vi "Run FGV Tests for 2D Double Array.vi"(2 "DELETE VI Reference":refnum<vi>, 3 "GET VI Reference":refnum<vi>, 4 "PUT VI Reference":refnum<vi>) -> (0 "Reason":string, 1 "Success":bool)   [LabVIEW 2013]
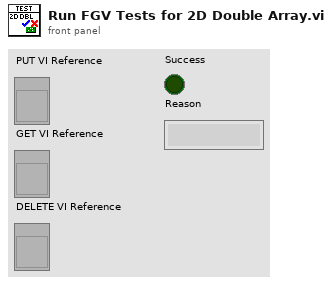
[diagram p1: front panel]
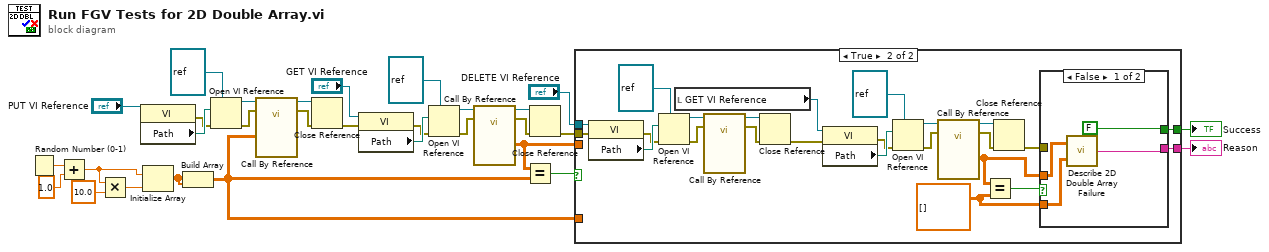
[diagram p0: block diagram]
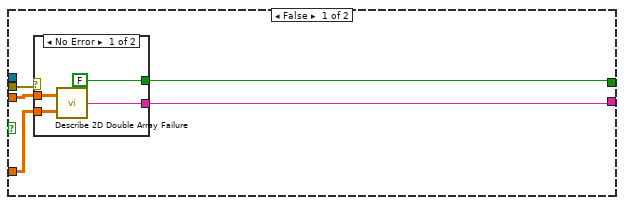
[diagram p2: hidden frame]
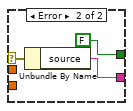
[diagram p3: hidden frame]
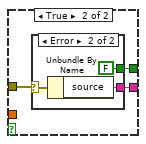
[diagram p4: hidden frame]
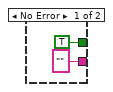
[diagram p5: hidden frame]
diagram:
  n1 = Random Number (0-1)() -> (number: 0 to 1=w15:dbl)
  n2 = Add(x=w15, y=1.0) -> (x+y=w3:dbl)
  n3 = Multiply(x=w3, y=10.0) -> (x*y=w4:dbl)
  n4 = property class="VI"(reference="PUT VI Reference") -> (error out=w8:errorcluster, "Path"=w21:path)  [unwired: 1 in, 1 out]
  n5 = Initialize Array(w3, w4) -> (w2:dbl[])
  n6 = Build Array(w2, w2) -> (w1:dbl[][])
  n7 = Open VI Reference(type specifier VI Refnum (for type only)=refnum<vi> refnum, vi path=w21, error in (no error)=w8) -> (vi reference=w20:refnum<vi>, error out=w19:errorcluster)  [unwired: 3 in]
  n8 = call-by-ref "?"(reference=w20, error in=w19, "Data"=w1) -> (reference out=w18:refnum<vi>, error out=w17:errorcluster)
  n9 = Close Reference(reference=w18, error in (no error)=w17) -> (error out=w13:errorcluster)
  n10 = property class="VI"(reference="GET VI Reference", error in=w13) -> (error out=w9:errorcluster, "Path"=w26:path)  [unwired: 1 out]
  n11 = Open VI Reference(type specifier VI Refnum (for type only)=refnum<vi> refnum, vi path=w26, error in (no error)=w9) -> (vi reference=w27:refnum<vi>, error out=w28:errorcluster)  [unwired: 3 in]
  n12 = call-by-ref "?"(reference=w27, error in=w28) -> (reference out=w29:refnum<vi>, error out=w30:errorcluster, "Data"=w10:dbl[][])
  n13 = Equal?(x=w10, y=w1) -> (x = y?=w11:bool)
  n14 = Close Reference(reference=w29, error in (no error)=w30) -> (error out=w12:errorcluster)
  n15 = case shown="True" w11 {
    tunnel: "DELETE VI Reference" -> [_ w60]
    tunnel: w12 -> [w31 w59]
    tunnel: w1 -> [w34 _]
    tunnel: w10 -> [w35 _]
    tunnel: [w33 w45] -> w7
    tunnel: [w32 w44] -> w6
    frame False {
      n16 = case shown="No Error" w31 {
        selector: w31 -> [_ w42]
        tunnel: w35 -> [w39 _]
        tunnel: w34 -> [w38 _]
        tunnel: [FALSE FALSE] -> w33
        tunnel: [w36 w40] -> w32
        frame No Error {
          n17 = call "Describe 2D Double Array Failure.vi"("Expected"=w38, "Got"=w39) -> ("Failure Description"=w36:string)
        }
        frame Error {
          n18 = Unbundle By Name(w42) -> ("source"=w40:string)
        }
      }
    }
    frame True {
      w43 = dbl[][] [] ("appended array")
      n19 = property class="VI"(reference=w60, error in=w59) -> (error out=w49:errorcluster, "Path"=w62:path)  [unwired: 1 out]
      n20 = Open VI Reference(type specifier VI Refnum (for type only)=refnum<vi> refnum, vi path=w62, error in (no error)=w49) -> (vi reference=w63:refnum<vi>, error out=w64:errorcluster)  [unwired: 3 in]
      n21 = local read "GET VI Reference"() -> (w47:refnum<vi>)
      n22 = call-by-ref "?"(reference=w63, error in=w64) -> (reference out=w65:refnum<vi>, error out=w66:errorcluster)  [unwired: 1 in]
      n23 = Close Reference(reference=w65, error in (no error)=w66) -> (error out=w52:errorcluster)
      n24 = property class="VI"(reference=w47, error in=w52) -> (error out=w50:errorcluster, "Path"=w54:path)  [unwired: 1 out]
      n25 = Open VI Reference(type specifier VI Refnum (for type only)=refnum<vi> refnum, vi path=w54, error in (no error)=w50) -> (vi reference=w55:refnum<vi>, error out=w56:errorcluster)  [unwired: 3 in]
      n26 = call-by-ref "?"(reference=w55, error in=w56) -> (reference out=w57:refnum<vi>, error out=w58:errorcluster, "Data"=w46:dbl[][])
      n27 = Equal?(x=w46, y=w43) -> (x = y?=w51:bool)
      n28 = Close Reference(reference=w57, error in (no error)=w58) -> (error out=w48:errorcluster)
      n29 = case shown="False" w51 {
        tunnel: w48 -> [_ w73]
        tunnel: w46 -> [w70 _]
        tunnel: w43 -> [w69 _]
        tunnel: [FALSE w72] -> w45
        tunnel: [w67 w71] -> w44
        frame False {
          n30 = call "Describe 2D Double Array Failure.vi"("Expected"=w69, "Got"=w70) -> ("Failure Description"=w67:string)
        }
        frame True {
          n31 = case shown="Error" w73 {
            selector: w73 -> [_ w78]
            tunnel: [TRUE FALSE] -> w72
            tunnel: ["" ("source") w76] -> w71
            frame No Error {
            }
            frame Error {
              n32 = Unbundle By Name(w78) -> ("source"=w76:string)
            }
          }
        }
      }
    }
  }
  "Success" <- w7
  "Reason" <- w6
